vi "RS485ReadSteamingOn.vi"() -> ()   [LabVIEW 2016]
uses:
  <vilib>/Instr/_visa.llb/VISA Set IO Buffer Mask.ctl
  <vilib>/Instr/_visa.llb/VISA Configure Serial Port (Instr).vi
panel:
  out "Array":i32[](array[numeric])
  out "#Valid Read":i32
  out "Total Time":dbl
  out "#Error":i32
  out "output array 2":dbl[](array[numeric])
  out "output array":dbl[](array[numeric])
  in  "VISA resource name":refnum<visa-resource-name>="COM4"
  in  "flow control":u16(ring) items=["None"=0, "XON/XOFF"=1, "RTS/CTS"=2, "DTR/DSR"=4]
  in  "stop bits":u16(ring)=10 items=["1"=10, "1.5"=15, "2.0"=20]
  in  "parity":u16(ring)=2 items=["None", "Odd", "Even", "Mark", "Space"]
  in  "data bits":u16=8 min=5 max=8 step=1
  in  "baud rate":u32=1500000
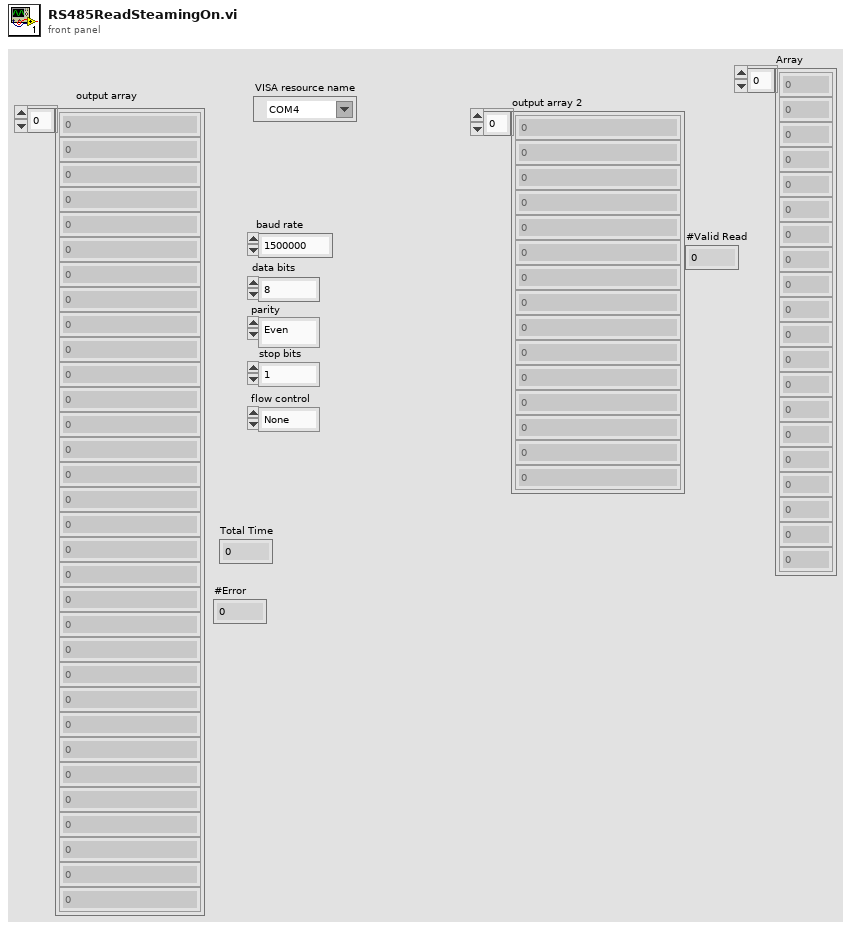
[diagram p1: front panel]
types:
  T1 = typedef "VISA Set IO Buffer Mask.ctl" = u16
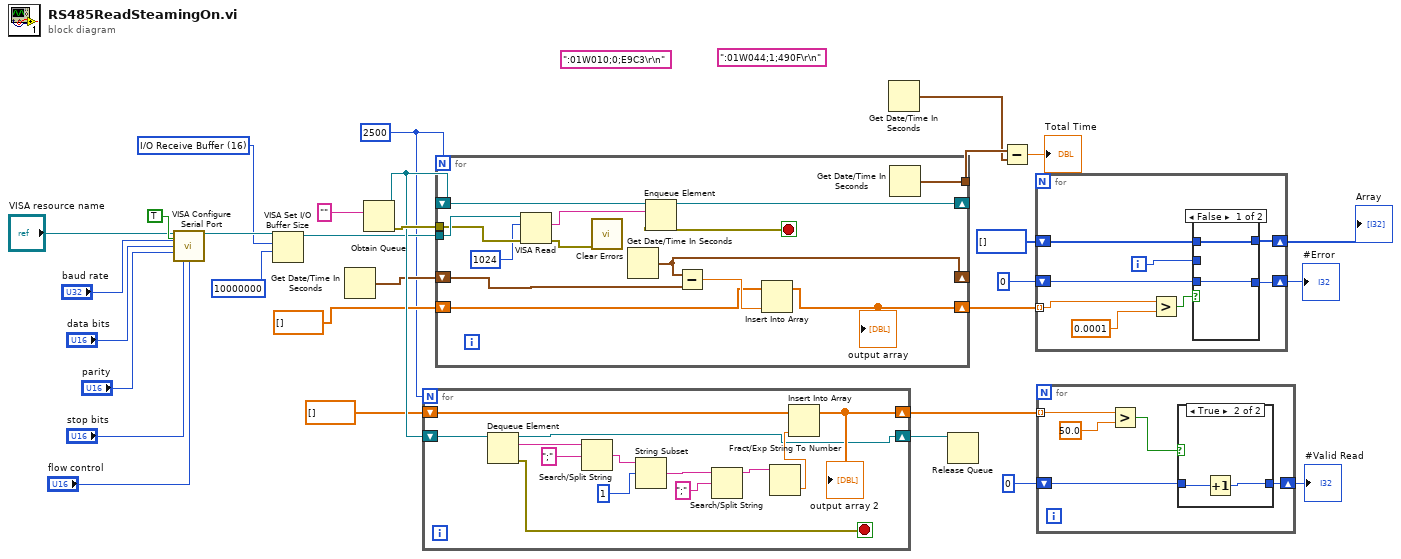
[diagram p0: block diagram]
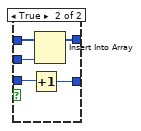
[diagram p3: hidden frame]
diagram:
  w10 = T1 16 items=["I/O Receive Buffer"=16, "I/O Transmit Buffer"=32, "I/O Receive and Transmit Buffer"=48] ("Mask")
  (unwired) ":01W010;0;E9C3\r\n" ("write buffer")
  (unwired) ":01W044;1;490F\r\n" ("write buffer")
  w9 = 2500
  n1 = call-poly "VISA Configure Serial Port"("VISA resource name"="VISA resource name", "Enable Termination\nChar (T)"=TRUE, "baud rate (9600)"="baud rate", "data bits (8)"="data bits", "parity (0:none)"="parity", "stop bits (10: 1 bit)"="stop bits", "flow control (0:none)"="flow control") -> ("VISA resource name out"=w16:refnum<visa-resource-name>)  [unwired: 7 in, 1 out]
  n2 = VISA Set I/O Buffer Size(VISA resource name=w16, mask (16)=w10, size (4096)=u32 10000000) -> (VISA resource name out=w15:refnum<visa-resource-name>)  [unwired: 1 in, 1 out]
  n3 = Get Date/Time In Seconds() -> (seconds since 1Jan1904=w20:timestamp)
  n4 = Obtain Queue(element data type="" ("write buffer")) -> (queue out=w21:refnum<queue>, error out=w22:errorcluster)  [unwired: 4 in, 1 out]
  n5 = for {
    N: w9 -> [_]
    shift-right: [w31] -> w17
    shift-left: w21 -> [w43]
    shift-right: [w33] -> w5
    shift-left: dbl[] [] -> [w34]
    stop <- w35 stop-if-true
    n6 = Dequeue Element(queue=w43) -> (queue out=w31:refnum<queue>, element=w36:string, error out=w35:errorcluster)  [unwired: 2 in, 1 out]
    n7 = Search/Split String(string=w36, search string/char (-)=";") -> (match + rest of string=w42:string)  [unwired: 1 in, 2 out]
    n8 = String Subset(string=w42, offset (0)=1) -> (substring=w39:string)  [unwired: 1 in]
    n9 = Search/Split String(string=w39, search string/char (-)=";") -> (substring before match=w41:string)  [unwired: 1 in, 2 out]
    n10 = Fract/Exp String To Number(string=w41) -> (number=w32:dbl)  [unwired: 3 in, 1 out]
    n11 = Insert Into Array(array=w34, new element=w32) -> (w33:dbl[])  [unwired: 1 in]
    "output array 2" <- w33
  }
  n12 = for {
    N: w9 -> [_]
    tunnel: w15 -> [w57]
    tunnel: w22 -> [w56]
    shift-right: [w54] -> _
    shift-left: w21 -> [w53]
    shift-right: [w50] -> _
    shift-left: w20 -> [w51]
    shift-right: [w47] -> w13
    shift-left: dbl[] [] -> [w48]
    tunnel: [w45] -> w8
    stop <- w52 stop-if-true
    n13 = VISA Read(VISA resource name=w57, byte count=u32 1024, error in (no error)=w56) -> (read buffer=w55:string, error out=w44:errorcluster)  [unwired: 2 out]
    n14 = call <vilib>:"Clear Errors.vi"("error in (no error)"=w44) -> ()  [unwired: 5 in, 2 out]
    n15 = Get Date/Time In Seconds() -> (seconds since 1Jan1904=w50:timestamp)
    n16 = Enqueue Element(queue=w53, element=w55) -> (queue out=w54:refnum<queue>, error out=w52:errorcluster)  [unwired: 2 in, 1 out]
    n17 = Subtract(x=w50, y=w51) -> (x-y=w49:dbl)
    n18 = Insert Into Array(array=w48, new element=w49) -> (w47:dbl[])  [unwired: 1 in]
    "output array" <- w47
    n19 = Get Date/Time In Seconds() -> (seconds since 1Jan1904=w45:timestamp)
  }
  n20 = Get Date/Time In Seconds() -> (seconds since 1Jan1904=w7:timestamp)
  n21 = Release Queue(queue=w17) -> ()  [unwired: 2 in, 3 out]
  n22 = Subtract(x=w8, y=w7) -> (x-y=→"Total Time":dbl)
  n23 = for {
    tunnel: w13 -> [w65] mode=indexing
    shift-right: [w61] -> w11
    shift-left: 0 -> [w62]
    shift-right: [w58] -> w1
    shift-left: i32[] [] -> [w60]
    i -> [w59]
    n24 = Greater?(x=w65, y=0.0001) -> (0:w63:bool)
    n25 = case shown="False" w63 {
      tunnel: w62 -> [w67 w72]
      tunnel: [w67 w71] -> w61
      tunnel: w60 -> [w66 w70]
      tunnel: w59 -> [_ w69]
      tunnel: [w66 w68] -> w58
      frame False {
      }
      frame True {
        n26 = Increment(x=w72) -> (x+1=w71:i32)
        n27 = Insert Into Array(array=w70, new element=w69) -> (w68:i32[])  [unwired: 1 in]
      }
    }
  }
  "#Error" <- w11
  "Array" <- w1
  n28 = for {
    tunnel: w5 -> [w77] mode=indexing
    shift-right: [w73] -> w3
    shift-left: 0 -> [w74]
    n29 = Greater?(x=w77, y=50.0) -> (0:w75:bool)
    n30 = case shown="True" w75 {
      tunnel: w74 -> [w78 w80]
      tunnel: [w78 w79] -> w73
      frame False {
      }
      frame True {
        n31 = Increment(x=w80) -> (x+1=w79:i32)
      }
    }
  }
  "#Valid Read" <- w3
